vi "Write Init_.vi"(8 "error in (no error)":errorcluster, 10 "Init?":bool, 11 "Avantes in":refnum<class "Avantes.lvclass">) -> (0 "error out":errorcluster, 3 "Avantes out":refnum<class "Avantes.lvclass">)   [LabVIEW 2020, in "Avantes.lvclass"]
uses:
  <instrlib>/Classes/CCD/Avantes/Avantes.lvclass
  <instrlib>/Classes/CCD/Avantes/Avantes.lvclass/Avantes.ctl
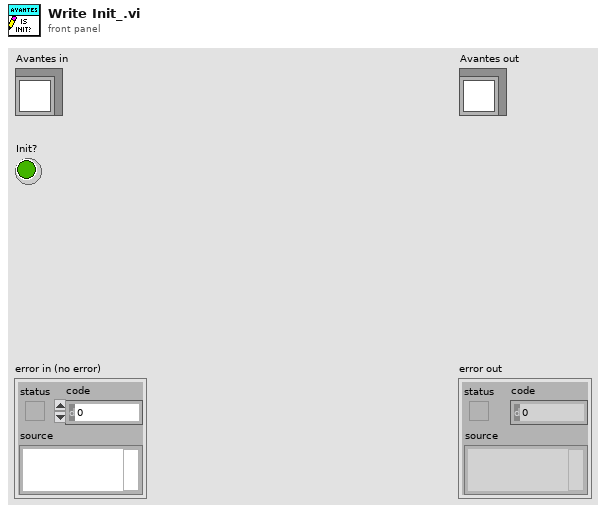
[diagram p1: front panel]
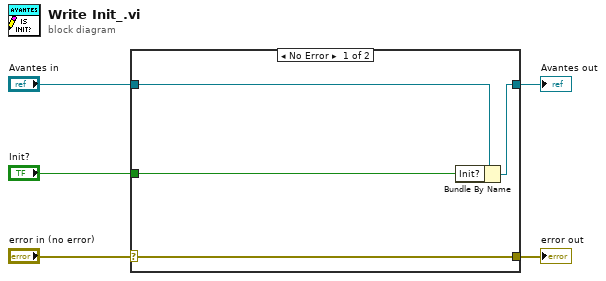
[diagram p0: block diagram]
diagram:
  n1 = case shown="No Error" "error in (no error)" {
    selector: "error in (no error)" -> [w9 w10]
    tunnel: [w9 w10] -> w4
    tunnel: [w7 w11] -> w2
    tunnel: "Avantes in" -> [w8 w11]
    tunnel: "Init?" -> [w6 _]
    frame No Error {
      n2 = Bundle By Name(cluster=w8, "Init?"=w6) -> (w7:refnum<class "Avantes.lvclass">)
    }
    frame Error {
    }
  }
  "error out" <- w4
  "Avantes out" <- w2
